vi "MotorPosition.vi"(3 "Motor":string="PI1-SHUTTER", 4 "Position":i32, 9 "error in (no error)":errorcluster) -> (0 "Motor out":string="PI1-SHUTTER", 6 "error out":errorcluster)   [LabVIEW 2009]
uses:
  Controls/MotorCommandBasic.ctl
  Controls/MotorCommand.ctl
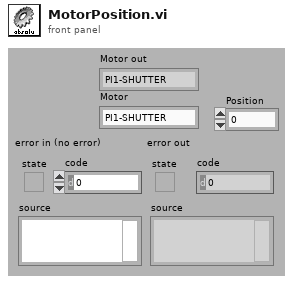
[diagram p1: front panel]
types:
  T1 = typedef "MotorStatus.ctl" = cluster{"Managed?":bool, "Position":i32, "Name":string, "Status":enum16{"OFF", "IDLE", "MOVING", "HOMING"}}
  T2 = typedef "MotorCommandBasic.ctl" = enum16{"SELECT", "MOVE", "PREMOVE", "TURBO", "POS", "NAMED", "INIT", "STOP", "OFF", "SPEED", "QUIT"}
  T3 = typedef "MotorCommand.ctl" = cluster{"Motor":string, "Command":T2, "Movement":i32, "Name":string, "Param":cluster{"VMIN":i32, "VMAX":i32, "ACC":i32}, "Ok?":refnum<k4>, "Go!":refnum<k4>}
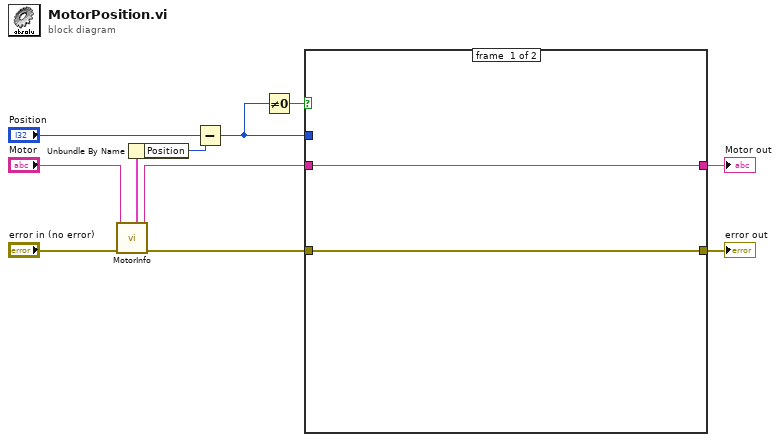
[diagram p0: block diagram]
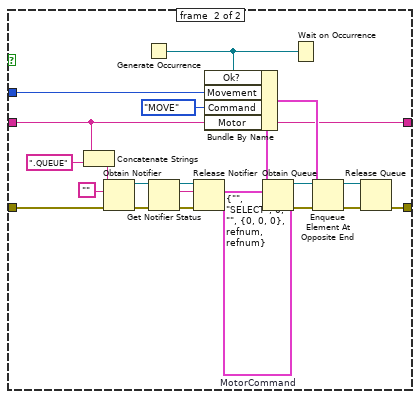
[diagram p2: hidden frame]
diagram:
  n1 = call "MotorInfo.vi"("error in (no error)"="error in (no error)", "Motor"="Motor") -> ("error out"=w9:errorcluster, "Motor out"=w7:string, "Axis status"=w6:T1)  [unwired: 5 out]
  n2 = Unbundle By Name(w6) -> ("Position"=w4:i32)
  n3 = Subtract(x="Position", y=w4) -> (x-y=w3:i32)
  n4 = Not Equal To 0?(x=w3) -> (x != 0?=w2:bool)
  n5 = case shown="True" w2 {
    tunnel: [w13 w19] -> w11
    tunnel: w9 -> [w13 w17]
    tunnel: w7 -> [w12 w14]
    tunnel: w3 -> [_ w15]
    tunnel: [w12 w14] -> w1
    frame #0 {
    }
    frame #1 {
      w32 = T3 {"Motor"="", "Command"=enum."SELECT", "Movement"=0, "Name"="", "Param"={"VMIN"=0, "VMAX"=0, "ACC"=0}, "Ok?"=refnum, "Go!"=refnum}  # MotorCommand
      n6 = Concatenate Strings(w14, ".QUEUE") -> (w23:string)
      n7 = Obtain Notifier(name (unnamed)=w23, notification data type="", error in (no error)=w17) -> (notifier out=w24:refnum<notifier>, error out=w25:errorcluster)  [unwired: 1 in, 1 out]
      n8 = Generate Occurrence() -> (w18:refnum<k4>)
      n9 = Get Notifier Status(notifier=w24, error in (no error)=w25) -> (notifier out=w27:refnum<notifier>, current notification=w20:string, error out=w28:errorcluster)  [unwired: 2 out]
      n10 = Release Notifier(notifier=w27, error in (no error)=w28) -> (error out=w21:errorcluster)  [unwired: 3 out]
      n11 = Bundle By Name(cluster=w32, "Ok?"=w18, "Movement"=w15, "Command"=MotorCommandBasic."MOVE", "Motor"=w14) -> (w31:T3)
      n12 = Obtain Queue(name (unnamed)=w20, element data type=w32, error in (no error)=w21) -> (queue out=w34:refnum<queue>, error out=w33:errorcluster)  [unwired: 2 in, 1 out]
      n13 = Wait on Occurrence(2:w18) -> ()  [unwired: 3 out]
      n14 = Enqueue Element At Opposite End(queue=w34, element=w31, error in (no error)=w33) -> (queue out=w29:refnum<queue>, error out=w30:errorcluster)  [unwired: 2 out]
      n15 = Release Queue(queue=w29, error in (no error)=w30) -> (error out=w19:errorcluster)  [unwired: 3 out]
    }
  }
  "error out" <- w11
  "Motor out" <- w1
